vi "Zoom in-out Graphs to mouse selection.vi"(10 "String":string, 11 "Data Cluster in":T1) -> (2 "Clear Graph ?":bool, 3 "Data Cluster out":T1)   [LabVIEW 2019, in "CML UI.lvlib"]
uses:
  CML UI.lvlib
  Module Data--cluster.ctl
  Acquisition State.ctl
  Measurement UI Displays.ctl
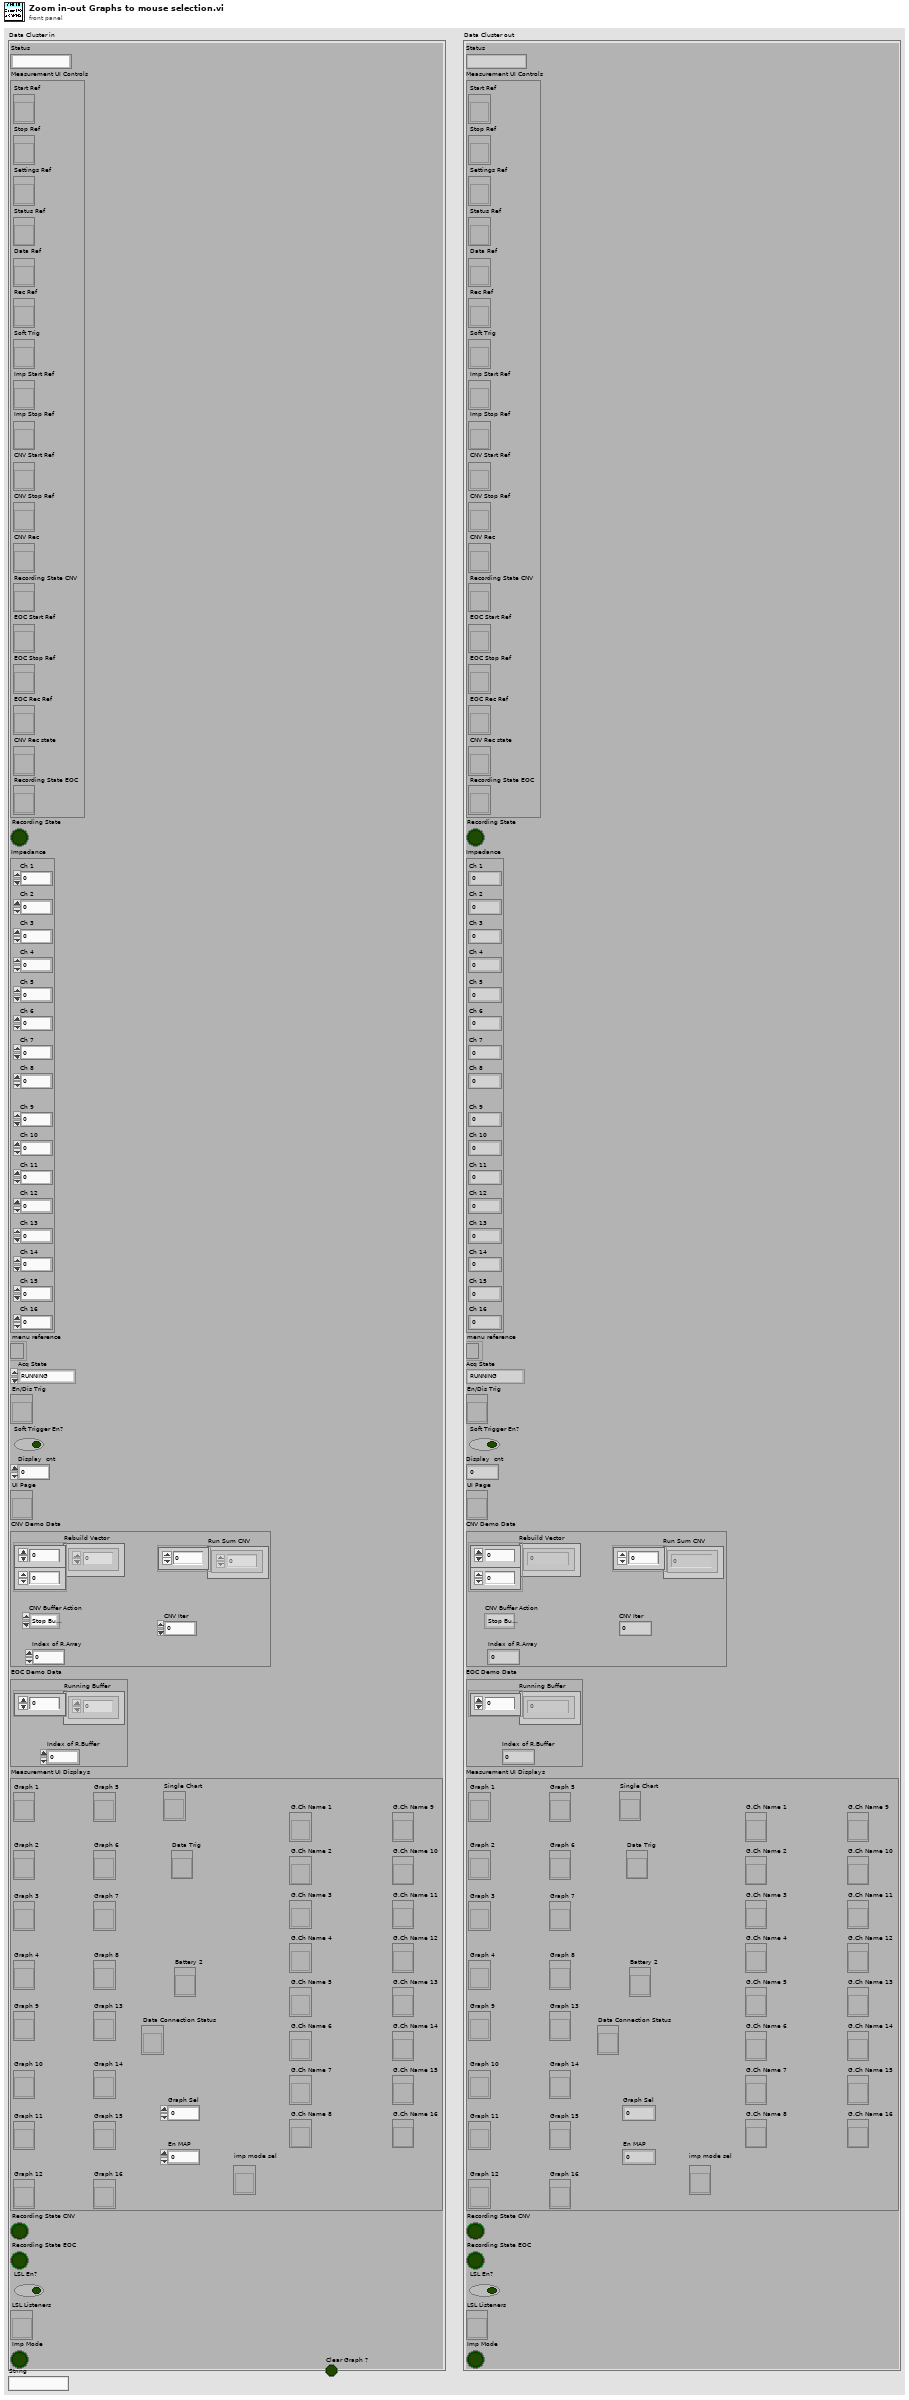
[diagram p1: front panel]
types:
  T1 = typedef "CML UI.lvlib/Module Data--cluster.ctl" = cluster{"Status":string, "Measurement UI Controls":cluster{"Start Ref":refnum<vi>, "Stop Ref":refnum<vi>, "Settings Ref":refnum<vi>, "Status Ref":refnum<vi>, "Data Ref":refnum<vi>, "Rec Ref":refnum<vi>, "Soft Trig":refnum<vi>, "Imp Start Ref":refnum<vi>, "Imp Stop Ref":refnum<vi>, "CNV Start Ref":refnum<vi>, "CNV Stop Ref":refnum<vi>, "CNV Rec":refnum<vi>, "Recording State CNV":refnum<vi>, "EOC Start Ref":refnum<vi>, "EOC Stop Ref":refnum<vi>, "EOC Rec Ref":refnum<vi>, "CNV Rec state":refnum<vi>, "Recording State EOC":refnum<vi>}, "Recording State":bool, "Impedance":cluster{"Ch 1":dbl, "Ch 2":dbl, "Ch 3":dbl, "Ch 4":dbl, "Ch 5":dbl, "Ch 6":dbl, "Ch 7":dbl, "Ch 8":dbl, "Ch 9":dbl, "Ch 10":dbl, "Ch 11":dbl, "Ch 12":dbl, "Ch 13":dbl, "Ch 14":dbl, "Ch 15":dbl, "Ch 16":dbl}, "menu reference ":refnum<k9>, "Acq State":T2, "En/Dis Trig":refnum<vi>, "Soft Trigger En?":bool, "Display  cnt":u8, "UI Page":refnum<vi>, "CNV Demo Data":cluster{"Rebuild Vector":dbl[][], "CNV Buffer Action":enum16{"Stop Buffer Fill", "Start Buffer Fill", "Analyze Buffer"}, "Index of R.Array":u16, "Run Sum CNV":dbl[], "CNV Iter":u16}, "EOC Demo Data":cluster{"Running Buffer":dbl[], "Index of R.Buffer":u8}, "Measurement UI Displays":T3, "Recording State CNV":bool, "Recording State EOC":bool, "LSL En?":bool, "LSL Listeners":refnum<vi>, "Imp Mode":bool}
  T2 = typedef "CML UI.lvlib/Acquisition State.ctl" = enum16{"RUNNING", "IDLE"}
  T3 = typedef "CML UI.lvlib/Measurement UI Displays.ctl" = cluster{"Graph 1":refnum<vi>, "Graph 2":refnum<vi>, "Graph 3":refnum<vi>, "Graph 4":refnum<vi>, "Graph 5":refnum<vi>, "Graph 6":refnum<vi>, "Graph 7":refnum<vi>, "Graph 8":refnum<vi>, "Graph 9":refnum<vi>, "Graph 10":refnum<vi>, "Graph 11":refnum<vi>, "Graph 12":refnum<vi>, "Graph 13":refnum<vi>, "Graph 14":refnum<vi>, "Graph 15":refnum<vi>, "Graph 16":refnum<vi>, "Battery 2":refnum<vi>, "Data Trig":refnum<vi>, "Data Connection Status":refnum<vi>, "Graph Sel":u8, "En MAP":u16, "Single Chart":refnum<vi>, "G.Ch Name 1":refnum<vi>, "G.Ch Name 2":refnum<vi>, "G.Ch Name 3":refnum<vi>, "G.Ch Name 4":refnum<vi>, "G.Ch Name 5":refnum<vi>, "G.Ch Name 6":refnum<vi>, "G.Ch Name 7":refnum<vi>, "G.Ch Name 8":refnum<vi>, "G.Ch Name 9":refnum<vi>, "G.Ch Name 10":refnum<vi>, "G.Ch Name 11":refnum<vi>, "G.Ch Name 12":refnum<vi>, "G.Ch Name 13":refnum<vi>, "G.Ch Name 14":refnum<vi>, "G.Ch Name 15":refnum<vi>, "G.Ch Name 16":refnum<vi>, "imp mode sel":refnum<vi>}
  T4 = enum32{"Graph", "Impedance", "More Options", "Single Graph", "CNV Demo", "Eyes O/C Demo"}
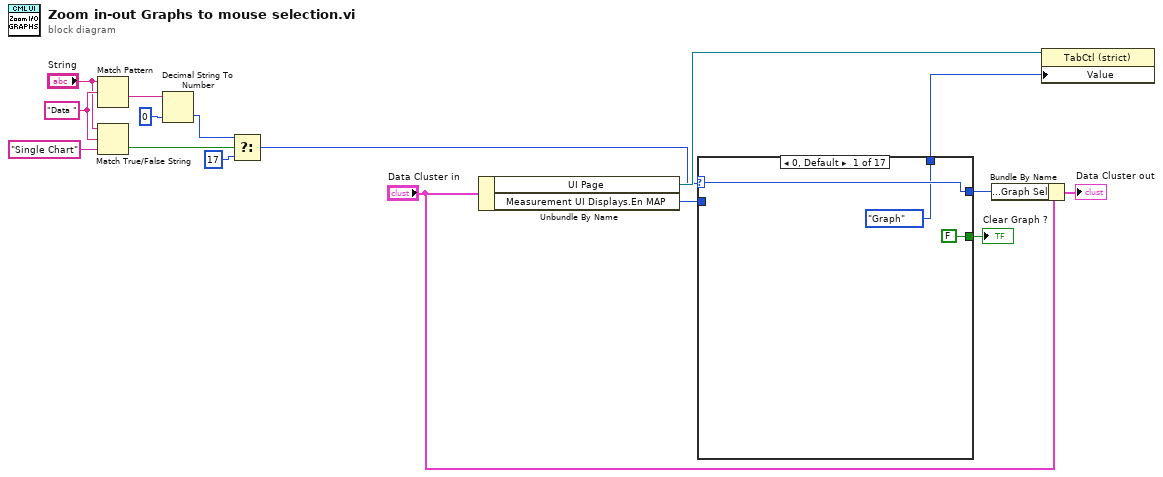
[diagram p0: block diagram]
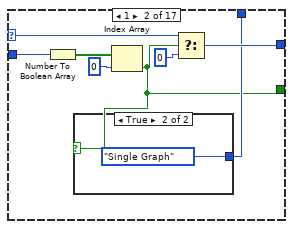
[diagram p2: hidden frame]
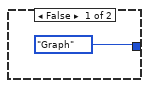
[diagram p3: hidden frame]
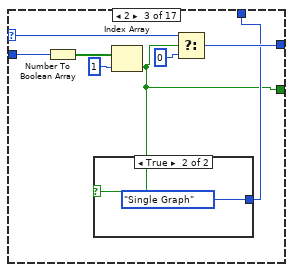
[diagram p4: hidden frame]
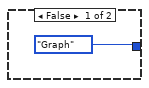
[diagram p5: hidden frame]
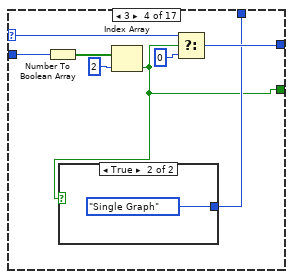
[diagram p6: hidden frame]
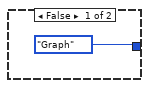
[diagram p7: hidden frame]
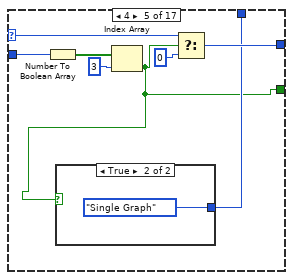
[diagram p8: hidden frame]
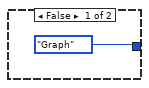
[diagram p9: hidden frame]
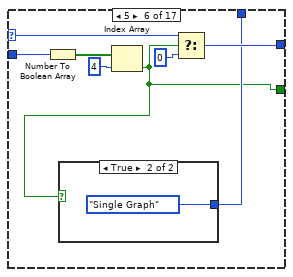
[diagram p10: hidden frame]
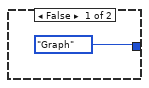
[diagram p11: hidden frame]
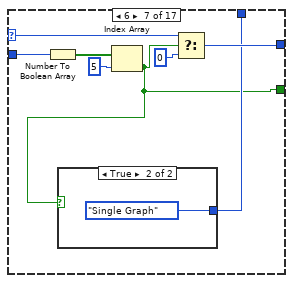
[diagram p12: hidden frame]
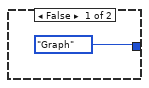
[diagram p13: hidden frame]
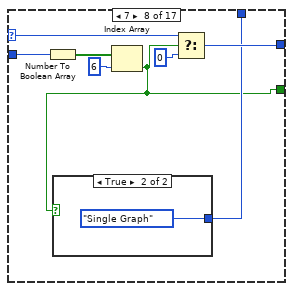
[diagram p14: hidden frame]
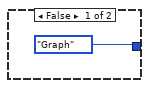
[diagram p15: hidden frame]
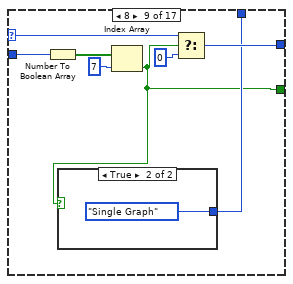
[diagram p16: hidden frame]
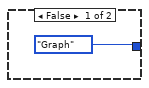
[diagram p17: hidden frame]
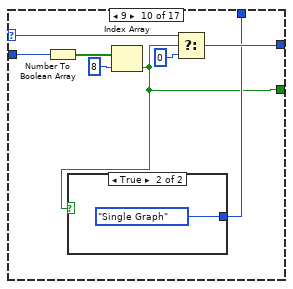
[diagram p18: hidden frame]
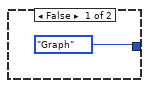
[diagram p19: hidden frame]
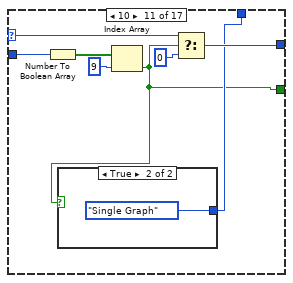
[diagram p20: hidden frame]
diagram:
  w9 = "Data " ("regular expression")
  n1 = Match Pattern(string="String", regular expression=w9) -> (after substring=w7:string)  [unwired: 1 in, 3 out]
  n2 = Match True/False String(2:"Single Chart" ("false string"), 3:w9, 4:"String") -> (0:w12:bool)  [unwired: 1 out]
  n3 = Decimal String To Number(string=w7, default (0L)=u8 0 ("default (0 I32)")) -> (number=w13:u8)  [unwired: 1 in, 1 out]
  n4 = Select(t=w13, s=w12, f=u8 17) -> (s? t:f=w3:u8)
  n5 = Unbundle By Name("Data Cluster in") -> ("UI Page"=w16:refnum<vi>, "Measurement UI Displays.En MAP"=w5:u16)
  n6 = case shown="0, Default" w3 {
    selector: w3 -> [w19 w24 w34 w44 w54 w64 w74 w84 w94 w104 w114 w124 w134 w144 w154 w164 w174]
    tunnel: w5 -> [_ w27 w37 w47 w57 w67 w77 w87 w97 w107 w117 w127 w137 w147 w157 w167 w177]
    tunnel: [w19 w22 w32 w42 w52 w62 w72 w82 w92 w102 w112 w122 w132 w142 w152 w162 w172] -> w4
    tunnel: [T4."Graph" ("Value") w21 w31 w41 w51 w61 w71 w81 w91 w101 w111 w121 w131 w141 w151 w161 w171] -> w2
    tunnel: [FALSE w20 w30 w40 w50 w60 w70 w80 w90 w100 w110 w120 w130 w140 w150 w160 w170] -> w1
    frame 0, Default {
    }
    frame 1 {
      n7 = Number To Boolean Array(number=w27) -> (Boolean array=w26:bool[])
      n8 = Index Array(array=w26, index=0) -> (element=w20:bool)
      n9 = case shown="True" w20 {
        tunnel: [T4."Graph" ("Value") T4."Single Graph" ("Value")] -> w21
        frame False {
        }
        frame True {
        }
      }
      n10 = Select(t=w24, s=w20, f=u8 0) -> (s? t:f=w22:u8)
    }
    frame 2 {
      n11 = Number To Boolean Array(number=w37) -> (Boolean array=w36:bool[])
      n12 = Index Array(array=w36, index=1) -> (element=w30:bool)
      n13 = case shown="True" w30 {
        tunnel: [T4."Graph" ("Value") T4."Single Graph" ("Value")] -> w31
        frame False {
        }
        frame True {
        }
      }
      n14 = Select(t=w34, s=w30, f=u8 0) -> (s? t:f=w32:u8)
    }
    frame 3 {
      n15 = Number To Boolean Array(number=w47) -> (Boolean array=w46:bool[])
      n16 = Index Array(array=w46, index=2) -> (element=w40:bool)
      n17 = case shown="True" w40 {
        tunnel: [T4."Graph" ("Value") T4."Single Graph" ("Value")] -> w41
        frame False {
        }
        frame True {
        }
      }
      n18 = Select(t=w44, s=w40, f=u8 0) -> (s? t:f=w42:u8)
    }
    frame 4 {
      n19 = Number To Boolean Array(number=w57) -> (Boolean array=w56:bool[])
      n20 = Index Array(array=w56, index=3) -> (element=w50:bool)
      n21 = case shown="True" w50 {
        tunnel: [T4."Graph" ("Value") T4."Single Graph" ("Value")] -> w51
        frame False {
        }
        frame True {
        }
      }
      n22 = Select(t=w54, s=w50, f=u8 0) -> (s? t:f=w52:u8)
    }
    frame 5 {
      n23 = Number To Boolean Array(number=w67) -> (Boolean array=w66:bool[])
      n24 = Index Array(array=w66, index=4) -> (element=w60:bool)
      n25 = case shown="True" w60 {
        tunnel: [T4."Graph" ("Value") T4."Single Graph" ("Value")] -> w61
        frame False {
        }
        frame True {
        }
      }
      n26 = Select(t=w64, s=w60, f=u8 0) -> (s? t:f=w62:u8)
    }
    frame 6 {
      n27 = Number To Boolean Array(number=w77) -> (Boolean array=w76:bool[])
      n28 = Index Array(array=w76, index=5) -> (element=w70:bool)
      n29 = case shown="True" w70 {
        tunnel: [T4."Graph" ("Value") T4."Single Graph" ("Value")] -> w71
        frame False {
        }
        frame True {
        }
      }
      n30 = Select(t=w74, s=w70, f=u8 0) -> (s? t:f=w72:u8)
    }
    frame 7 {
      n31 = Number To Boolean Array(number=w87) -> (Boolean array=w86:bool[])
      n32 = Index Array(array=w86, index=6) -> (element=w80:bool)
      n33 = case shown="True" w80 {
        tunnel: [T4."Graph" ("Value") T4."Single Graph" ("Value")] -> w81
        frame False {
        }
        frame True {
        }
      }
      n34 = Select(t=w84, s=w80, f=u8 0) -> (s? t:f=w82:u8)
    }
    frame 8 {
      n35 = Number To Boolean Array(number=w97) -> (Boolean array=w96:bool[])
      n36 = Index Array(array=w96, index=7) -> (element=w90:bool)
      n37 = case shown="True" w90 {
        tunnel: [T4."Graph" ("Value") T4."Single Graph" ("Value")] -> w91
        frame False {
        }
        frame True {
        }
      }
      n38 = Select(t=w94, s=w90, f=u8 0) -> (s? t:f=w92:u8)
    }
    frame 9 {
      n39 = Number To Boolean Array(number=w107) -> (Boolean array=w106:bool[])
      n40 = Index Array(array=w106, index=8) -> (element=w100:bool)
      n41 = case shown="True" w100 {
        tunnel: [T4."Graph" ("Value") T4."Single Graph" ("Value")] -> w101
        frame False {
        }
        frame True {
        }
      }
      n42 = Select(t=w104, s=w100, f=u8 0) -> (s? t:f=w102:u8)
    }
    frame 10 {
      n43 = Number To Boolean Array(number=w117) -> (Boolean array=w116:bool[])
      n44 = Index Array(array=w116, index=9) -> (element=w110:bool)
      n45 = case shown="True" w110 {
        tunnel: [T4."Graph" ("Value") T4."Single Graph" ("Value")] -> w111
        frame False {
        }
        frame True {
        }
      }
      n46 = Select(t=w114, s=w110, f=u8 0) -> (s? t:f=w112:u8)
    }
    frame 11 {
      n47 = Number To Boolean Array(number=w127) -> (Boolean array=w126:bool[])
      n48 = Index Array(array=w126, index=10) -> (element=w120:bool)
      n49 = case shown="True" w120 {
        tunnel: [T4."Graph" ("Value") T4."Single Graph" ("Value")] -> w121
        frame False {
        }
        frame True {
        }
      }
      n50 = Select(t=w124, s=w120, f=u8 0) -> (s? t:f=w122:u8)
    }
    frame 12 {
      n51 = Number To Boolean Array(number=w137) -> (Boolean array=w136:bool[])
      n52 = Index Array(array=w136, index=11) -> (element=w130:bool)
      n53 = case shown="True" w130 {
        tunnel: [T4."Graph" ("Value") T4."Single Graph" ("Value")] -> w131
        frame False {
        }
        frame True {
        }
      }
      n54 = Select(t=w134, s=w130, f=u8 0) -> (s? t:f=w132:u8)
    }
    frame 13 {
      n55 = Number To Boolean Array(number=w147) -> (Boolean array=w146:bool[])
      n56 = Index Array(array=w146, index=12) -> (element=w140:bool)
      n57 = case shown="True" w140 {
        tunnel: [T4."Graph" ("Value") T4."Single Graph" ("Value")] -> w141
        frame False {
        }
        frame True {
        }
      }
      n58 = Select(t=w144, s=w140, f=u8 0) -> (s? t:f=w142:u8)
    }
    frame 14 {
      n59 = Number To Boolean Array(number=w157) -> (Boolean array=w156:bool[])
      n60 = Index Array(array=w156, index=13) -> (element=w150:bool)
      n61 = case shown="True" w150 {
        tunnel: [T4."Graph" ("Value") T4."Single Graph" ("Value")] -> w151
        frame False {
        }
        frame True {
        }
      }
      n62 = Select(t=w154, s=w150, f=u8 0) -> (s? t:f=w152:u8)
    }
    frame 15 {
      n63 = Number To Boolean Array(number=w167) -> (Boolean array=w166:bool[])
      n64 = Index Array(array=w166, index=14) -> (element=w160:bool)
      n65 = case shown="True" w160 {
        tunnel: [T4."Graph" ("Value") T4."Single Graph" ("Value")] -> w161
        frame False {
        }
        frame True {
        }
      }
      n66 = Select(t=w164, s=w160, f=u8 0) -> (s? t:f=w162:u8)
    }
    frame 16 {
      n67 = Number To Boolean Array(number=w177) -> (Boolean array=w176:bool[])
      n68 = Index Array(array=w176, index=15) -> (element=w170:bool)
      n69 = case shown="True" w170 {
        tunnel: [T4."Graph" ("Value") T4."Single Graph" ("Value")] -> w171
        frame False {
        }
        frame True {
        }
      }
      n70 = Select(t=w174, s=w170, f=u8 0) -> (s? t:f=w172:u8)
    }
  }
  "Clear Graph ?" <- w1
  n71 = Bundle By Name(cluster="Data Cluster in", "Measurement UI Displays.Graph Sel"=w4) -> (→"Data Cluster out":T1)
  n72 = property class="TabCtl (strict)"(reference=w16, "Value"=w2) -> ()  [unwired: 1 in, 2 out]
